vi "Equations.vi"() -> ()   [LabVIEW 2020]
panel:
  out "x2":dbl=-5.0
  out "x1":dbl=3.0
  in  "c":dbl=-15.0
  in  "b":dbl=2.0
  in  "a":dbl=1.0
  out "Area":dbl=47882219803.87908
  in  "Radius of Circle":dbl=123456.0
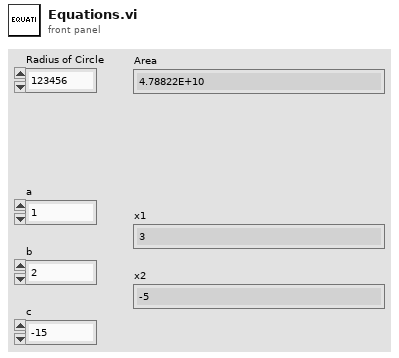
[diagram p1: front panel]
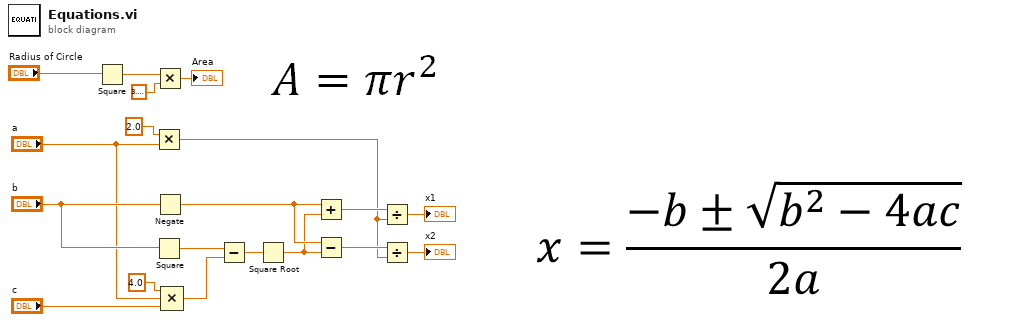
[diagram p0: block diagram]
diagram:
  n1 = Square(x="Radius of Circle") -> (x^2=w4:dbl)
  n2 = Multiply(x=2.0, y="a") -> (x*y=w6:dbl)
  n3 = Square(x="b") -> (x^2=w14:dbl)
  n4 = Multiply(x=w4, y=3.141592653589793) -> (x*y=→"Area":dbl)
  n5 = Negate(x="b") -> (-x=w9:dbl)
  n6 = Compound Arithmetic op=MULTIPLY(4.0, "a", "c") -> (w13:dbl)
  n7 = Subtract(x=w14, y=w13) -> (x-y=w12:dbl)
  n8 = Square Root(x=w12) -> (sqrt(x)=w8:dbl)
  n9 = Add(x=w9, y=w8) -> (x+y=w11:dbl)
  n10 = Subtract(x=w9, y=w8) -> (x-y=w7:dbl)
  n11 = Divide(x=w11, y=w6) -> (x/y=→"x1":dbl)
  n12 = Divide(x=w7, y=w6) -> (x/y=→"x2":dbl)
